vi "AlAs_GaAs_wait_SL_1.vi"(2 "Debug Mode":bool, 3 "Elapsed Time(s)":dbl, 4 "State":enum16{"Edit", "Start", "Run", "End", "Idle"}(ring), 5 "Argument List In":string[](array[string])) -> (0 "Status Out":string, 1 "Argument List Out":string[](array[string]))   [LabVIEW 2011]
doc: "This VI oscillates the flow of Gallium in a square wave according to the \"Period\" and \"Amplitude\" parameters. See the API Programming Guide for more details."
panel:
  in  "tWait2(s)":dbl
  in  "tWait1(s)":dbl
  out "tPeriod(s)":dbl
  in  "periods":dbl
  in  "tGa (s)":dbl
  in  "Ga flow (sccm)":dbl
  in  "tAl (s)":dbl
  in  "Al flow (sccm)":dbl
  in  "Cancel":bool
  in  "OK":bool
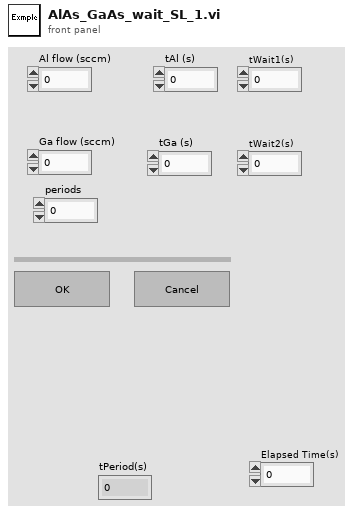
[diagram p1: front panel]
types:
  T1 = enum16{"Discrete", "Continuous", "Instantaneous"}
  T2 = enum32{"Invalid", "Default", "Floating", "Floating/Auto-Hide", "Modal"}
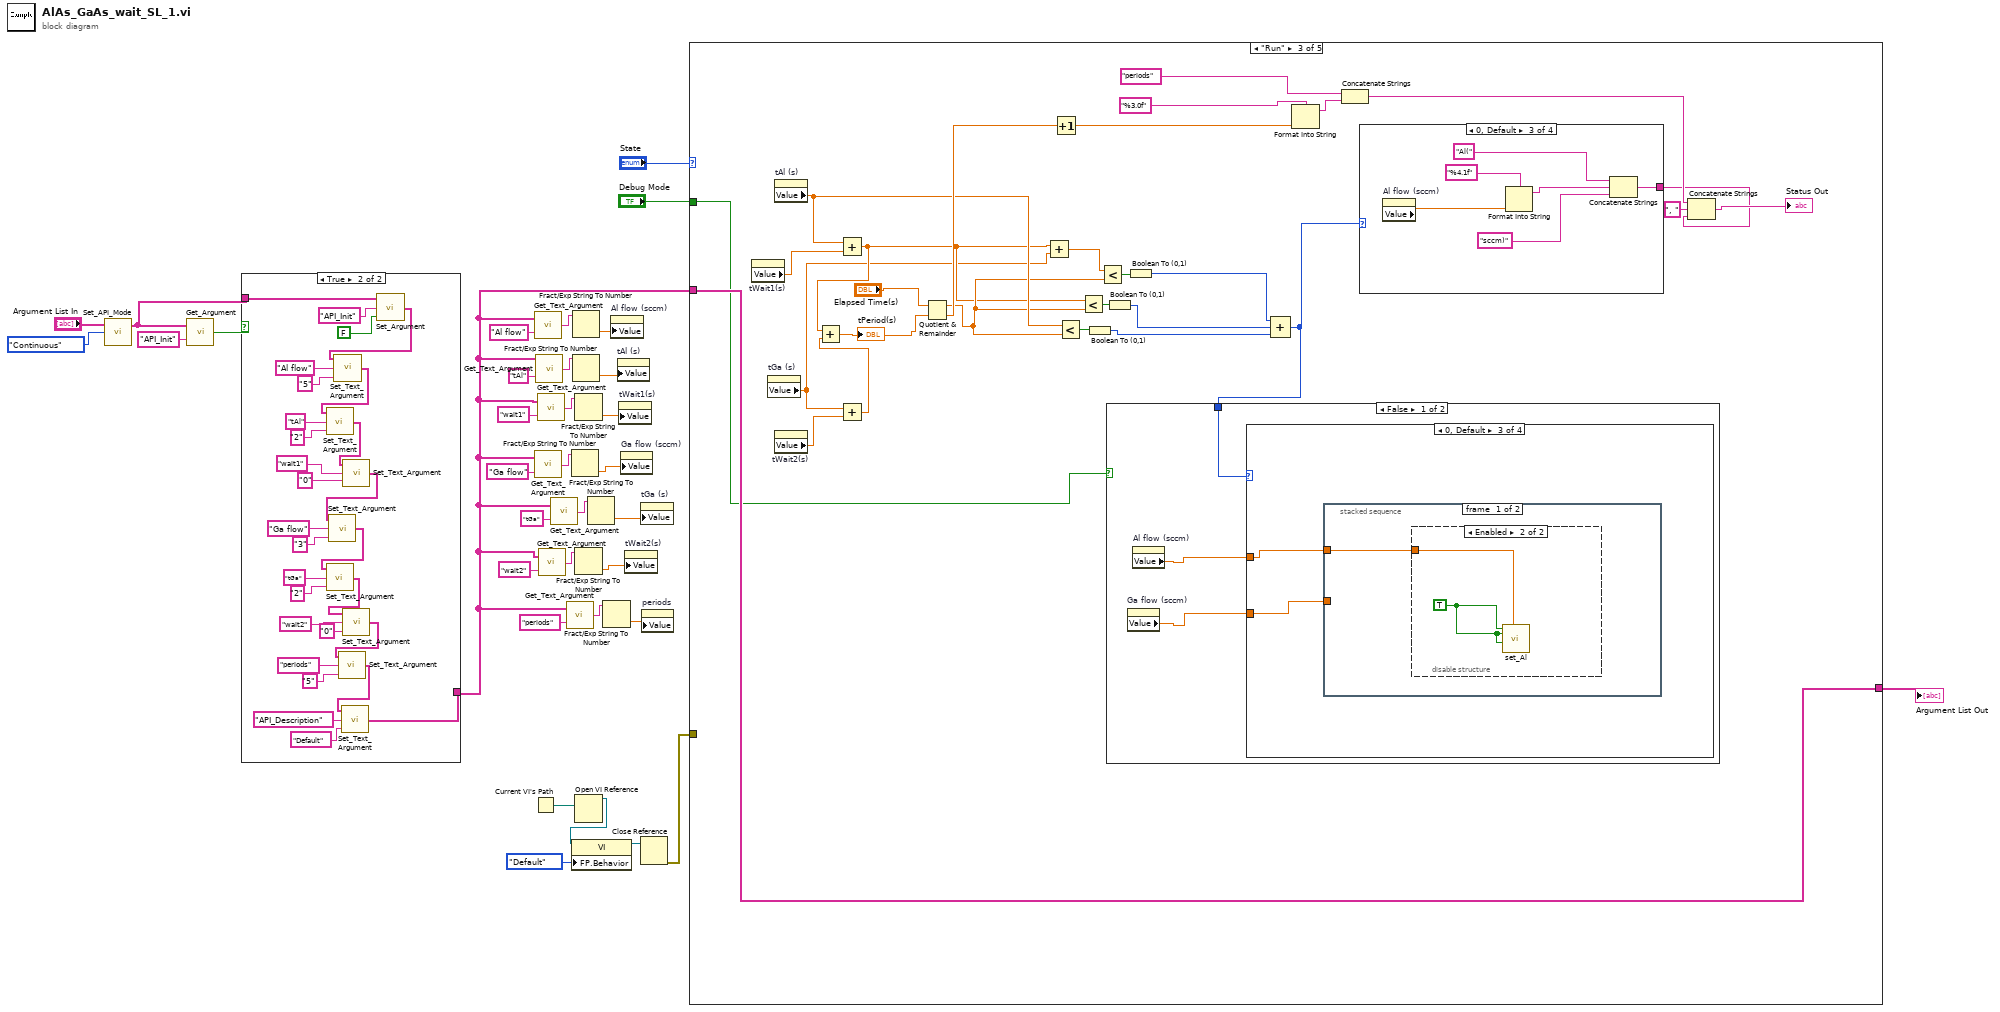
[diagram p0: block diagram]
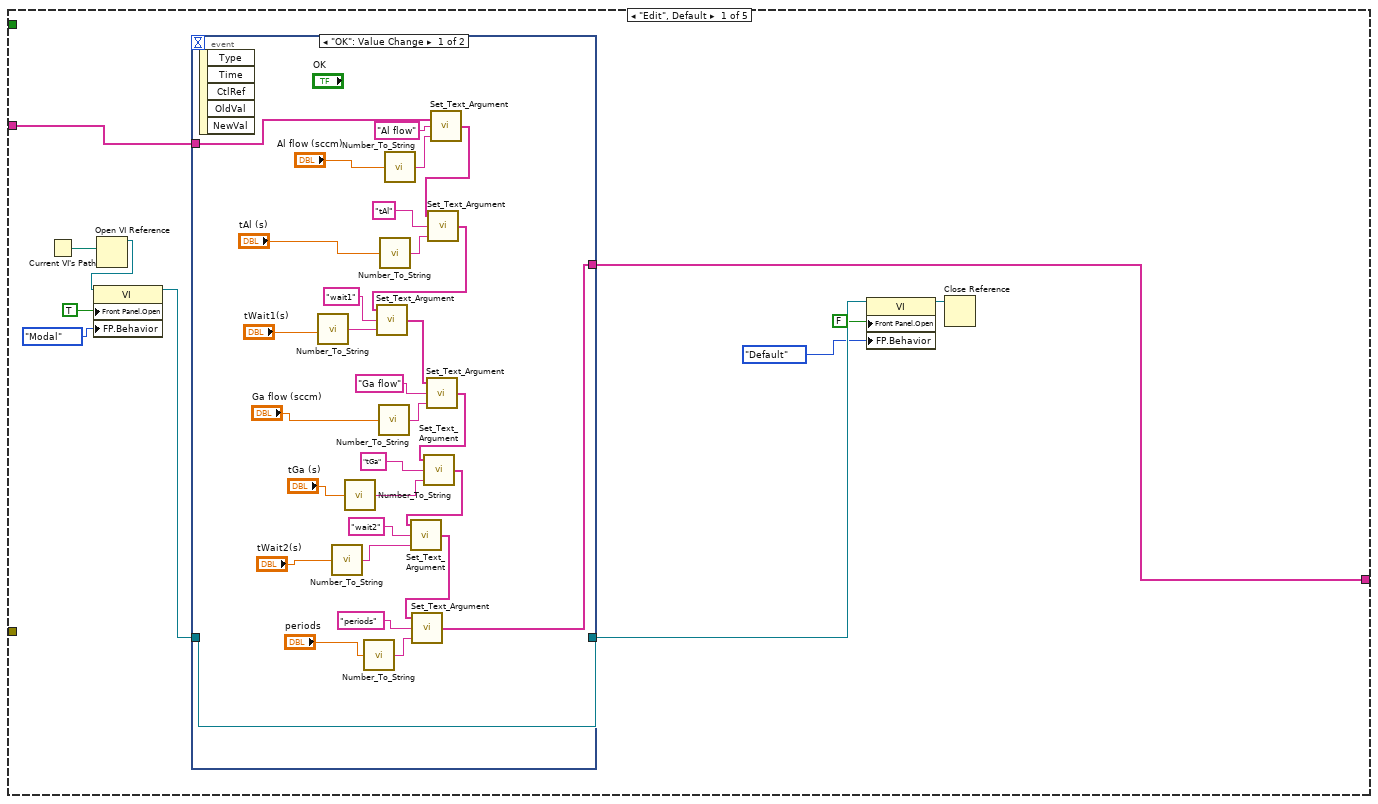
[diagram p3: hidden frame]
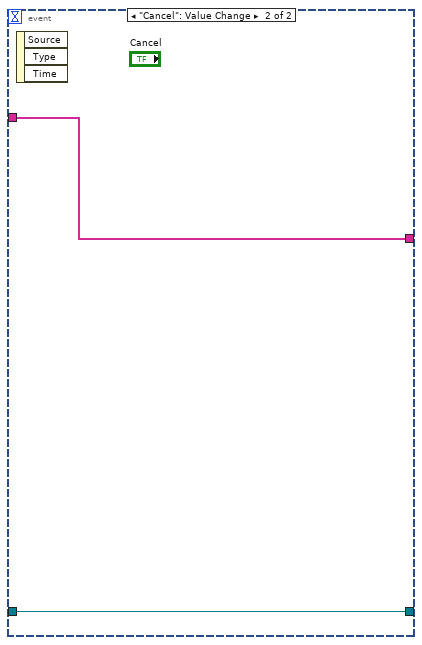
[diagram p4: hidden frame]
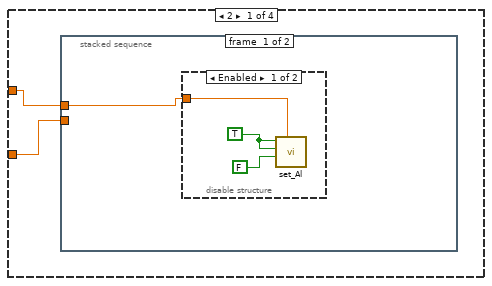
[diagram p6: hidden frame]
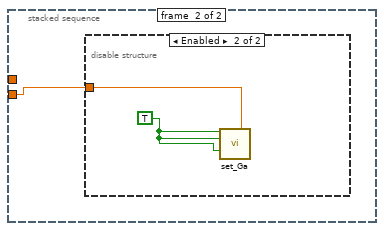
[diagram p8: hidden frame]
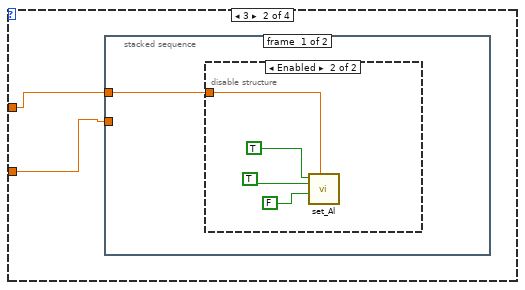
[diagram p10: hidden frame]
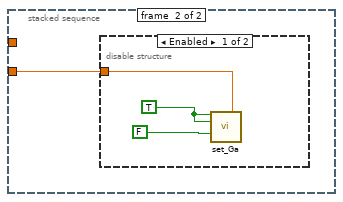
[diagram p12: hidden frame]
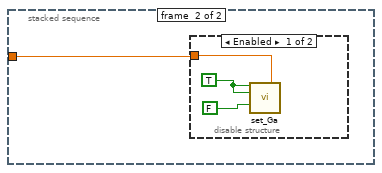
[diagram p15: hidden frame]
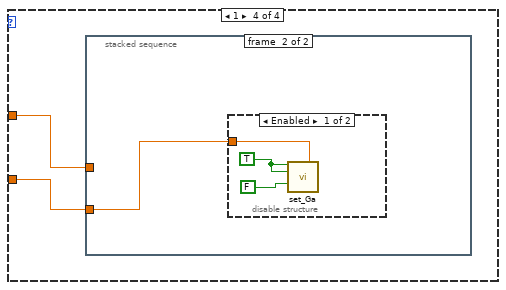
[diagram p17: hidden frame]
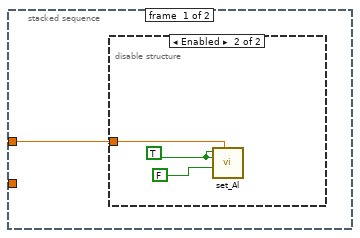
[diagram p18: hidden frame]
diagram:
  n1 = call "Set_API_Mode.vi"("API Mode"=T1."Continuous", "Argument List In"="Argument List In") -> ("Argument List Out"=w22:string[])  [unwired: 2 out]
  n2 = call "Get_Argument.vi"("Argument"="API_Init", "Argument List"=w22) -> ("Enabled"=w23:bool)
  n3 = case shown="True" w23 {
    tunnel: w22 -> [w36 w64]
    tunnel: [w36 w60] -> w3
    frame False {
    }
    frame True {
      n4 = call "Set_Argument.vi"("Enable"=FALSE, "Argument"="API_Init", "Argument List In"=w64) -> ("Argument List Out"=w45:string[])
      n5 = call "Set_Text_Argument.vi"("Text"="5", "Argument"="Al flow", "Argument List In"=w45) -> ("Argument List Out"=w46:string[])
      n6 = call "Set_Text_Argument.vi"("Text"="2", "Argument"="tAl", "Argument List In"=w46) -> ("Argument List Out"=w42:string[])
      n7 = call "Set_Text_Argument.vi"("Text"="0", "Argument"="wait1", "Argument List In"=w42) -> ("Argument List Out"=w41:string[])
      n8 = call "Set_Text_Argument.vi"("Text"="3", "Argument"="Ga flow", "Argument List In"=w41) -> ("Argument List Out"=w47:string[])
      n9 = call "Set_Text_Argument.vi"("Text"="2", "Argument"="tGa", "Argument List In"=w47) -> ("Argument List Out"=w44:string[])
      n10 = call "Set_Text_Argument.vi"("Text"="0", "Argument"="wait2", "Argument List In"=w44) -> ("Argument List Out"=w43:string[])
      n11 = call "Set_Text_Argument.vi"("Text"="5", "Argument"="periods", "Argument List In"=w43) -> ("Argument List Out"=w48:string[])
      n12 = call "Set_Text_Argument.vi"("Text"="Default", "Argument"="API_Description", "Argument List In"=w48) -> ("Argument List Out"=w60:string[])
    }
  }
  n13 = Current VI's Path() -> (path=w31:path)
  n14 = call "Get_Text_Argument.vi"("Argument"="Al flow", "Argument List"=w3) -> ("Text"=w20:string)
  n15 = call "Get_Text_Argument.vi"("Argument"="Ga flow", "Argument List"=w3) -> ("Text"=w17:string)
  n16 = call "Get_Text_Argument.vi"("Argument"="tAl", "Argument List"=w3) -> ("Text"=w19:string)
  n17 = call "Get_Text_Argument.vi"("Argument"="wait1", "Argument List"=w3) -> ("Text"=w6:string)
  n18 = call "Get_Text_Argument.vi"("Argument"="wait2", "Argument List"=w3) -> ("Text"=w2:string)
  n19 = call "Get_Text_Argument.vi"("Argument"="tGa", "Argument List"=w3) -> ("Text"=w15:string)
  n20 = call "Get_Text_Argument.vi"("Argument"="periods", "Argument List"=w3) -> ("Text"=w13:string)
  n21 = Fract/Exp String To Number(string=w17) -> (number=w10:dbl)  [unwired: 4 out]
  n22 = Fract/Exp String To Number(string=w20) -> (number=w12:dbl)  [unwired: 4 out]
  n23 = Fract/Exp String To Number(string=w19) -> (number=w11:dbl)  [unwired: 4 out]
  n24 = Fract/Exp String To Number(string=w6) -> (number=w5:dbl)  [unwired: 4 out]
  n25 = Fract/Exp String To Number(string=w2) -> (number=w1:dbl)  [unwired: 4 out]
  n26 = Open VI Reference(vi path=w31) -> (vi reference=w30:refnum<vi>)  [unwired: 1 in, 5 out]
  n27 = property class="VI"(reference=w30, "FP.Behavior"=T2."Default" ("Front Panel Window:Behavior")) -> (reference out=w28:refnum<vi>)  [unwired: 1 in, 1 out]
  n28 = Fract/Exp String To Number(string=w15) -> (number=w9:dbl)  [unwired: 4 out]
  n29 = Fract/Exp String To Number(string=w13) -> (number=w8:dbl)  [unwired: 4 out]
  n30 = property on="Al flow (sccm)" class="DigNum (strict)"("Value"=w12) -> ()  [unwired: 2 in, 2 out]
  n31 = property on="tAl (s)" class="DigNum (strict)"("Value"=w11) -> ()  [unwired: 2 in, 2 out]
  n32 = property on="tWait1(s)" class="DigNum (strict)"("Value"=w5) -> ()  [unwired: 2 in, 2 out]
  n33 = property on="Ga flow (sccm)" class="DigNum (strict)"("Value"=w10) -> ()  [unwired: 2 in, 2 out]
  n34 = property on="tWait2(s)" class="DigNum (strict)"("Value"=w1) -> ()  [unwired: 2 in, 2 out]
  n35 = property on="tGa (s)" class="DigNum (strict)"("Value"=w9) -> ()  [unwired: 2 in, 2 out]
  n36 = Close Reference(reference=w28) -> (error out=w27:errorcluster)  [unwired: 1 in]
  n37 = property on="periods" class="DigNum (strict)"("Value"=w8) -> ()  [unwired: 2 in, 2 out]
  n38 = case shown="\"Run\"" "State" {
    tunnel: [w75 w108 w136 w194 w195] -> w34
    tunnel: w3 -> [w74 w108 w136 w194 w195]
    tunnel: "Debug Mode" -> [_ _ w110 w193 _]
    tunnel: w27 -> [_ _ _ _ _]
    frame "Edit", Default {
      n39 = Current VI's Path() -> (path=w69:path)
      n40 = Open VI Reference(vi path=w69) -> (vi reference=w68:refnum<vi>)  [unwired: 1 in, 5 out]
      n41 = property class="VI"(reference=w68, "Front Panel.Open"=TRUE ("Front Panel Window:Open"), "FP.Behavior"=T2."Modal" ("Front Panel Window:Behavior")) -> (reference out=w72:refnum<vi>)  [unwired: 1 in, 1 out]
      n42 = event shown="[0] \"OK\": Value Change" {
        selector: _ -> [_ _]
        dyn-events: _ -> [_ _]
        timeout: _ -> [_ _]
        tunnel: w74 -> [w100 w106]
        tunnel: [w90 w106] -> w75
        tunnel: [w104 w107] -> w71
        tunnel: w72 -> [w104 w107]
        event "OK": Value Change {
          n43 = event-data() -> ()  [unwired: 6 out]
          n44 = call "Number_To_String.vi"("Number"="tWait1(s)") -> ("String"=w85:string)
          n45 = call "Number_To_String.vi"("Number"="tWait2(s)") -> ("String"=w79:string)
          n46 = call "Number_To_String.vi"("Number"="tGa (s)") -> ("String"=w94:string)
          n47 = call "Number_To_String.vi"("Number"="periods") -> ("String"=w92:string)
          n48 = call "Number_To_String.vi"("Number"="Ga flow (sccm)") -> ("String"=w96:string)
          n49 = call "Number_To_String.vi"("Number"="tAl (s)") -> ("String"=w101:string)
          n50 = call "Number_To_String.vi"("Number"="Al flow (sccm)") -> ("String"=w97:string)
          n51 = call "Set_Text_Argument.vi"("Text"=w97, "Argument"="Al flow" ("Text"), "Argument List In"=w100) -> ("Argument List Out"=w102:string[])
          n52 = call "Set_Text_Argument.vi"("Text"=w101, "Argument"="tAl", "Argument List In"=w102) -> ("Argument List Out"=w83:string[])
          n53 = call "Set_Text_Argument.vi"("Text"=w85, "Argument"="wait1", "Argument List In"=w83) -> ("Argument List Out"=w82:string[])
          n54 = call "Set_Text_Argument.vi"("Text"=w96, "Argument"="Ga flow", "Argument List In"=w82) -> ("Argument List Out"=w88:string[])
          n55 = call "Set_Text_Argument.vi"("Text"=w94, "Argument"="tGa", "Argument List In"=w88) -> ("Argument List Out"=w81:string[])
          n56 = call "Set_Text_Argument.vi"("Text"=w79, "Argument"="wait2", "Argument List In"=w81) -> ("Argument List Out"=w80:string[])
          n57 = call "Set_Text_Argument.vi"("Text"=w92, "Argument"="periods", "Argument List In"=w80) -> ("Argument List Out"=w90:string[])
        }
        event "Cancel": Value Change {
          n58 = event-data() -> ()  [unwired: 4 out]
        }
      }
      n59 = property class="VI"(reference=w71, "Front Panel.Open"=FALSE ("Front Panel Window:Open"), "FP.Behavior"=T2."Default" ("Front Panel Window:Behavior")) -> (reference out=w65:refnum<vi>)  [unwired: 1 in, 1 out]
      n60 = Close Reference(reference=w65) -> ()  [unwired: 1 in, 1 out]
    }
    frame "Start" {
    }
    frame "Run" {
      n61 = property on="tWait1(s)" class="DigNum (strict)"() -> ("Value"=w111:dbl)  [unwired: 2 in, 2 out]
      n62 = property on="tGa (s)" class="DigNum (strict)"() -> ("Value"=w121:dbl)  [unwired: 2 in, 2 out]
      n63 = property on="tAl (s)" class="DigNum (strict)"() -> ("Value"=w124:dbl)  [unwired: 2 in, 2 out]
      n64 = property on="tWait2(s)" class="DigNum (strict)"() -> ("Value"=w112:dbl)  [unwired: 2 in, 2 out]
      n65 = Add(x=w124, y=w111) -> (x+y=w122:dbl)
      n66 = Add(x=w121, y=w112) -> (x+y=w125:dbl)
      n67 = Add(x=w122, y=w125) -> (x+y=w127:dbl)
      "tPeriod(s)" <- w127
      n68 = Quotient & Remainder(x="Elapsed Time(s)", y=w127) -> (x-y*floor(x/y)=w123:dbl, floor(x/y)=w126:dbl)
      n69 = Add(x=w122, y=w121) -> (x+y=w120:dbl)
      n70 = Increment(x=w126) -> (x+1=w132:dbl)
      n71 = Less?(x=w124, y=w123) -> (x < y?=w119:bool)
      n72 = Less?(x=w122, y=w123) -> (x < y?=w117:bool)
      n73 = Boolean To (0,1)(Boolean=w119) -> (0, 1=w118:i16)
      n74 = Less?(x=w120, y=w123) -> (x < y?=w115:bool)
      n75 = Boolean To (0,1)(Boolean=w117) -> (0, 1=w116:i16)
      n76 = Boolean To (0,1)(Boolean=w115) -> (0, 1=w114:i16)
      n77 = Compound Arithmetic op=ADD(w114, w116, w118) -> (w109:i16)
      n78 = case shown="False" w110 {
        tunnel: w109 -> [w139 _]
        frame False {
          n79 = property on="Ga flow (sccm)" class="DigNum (strict)"() -> ("Value"=w137:dbl)  [unwired: 2 in, 2 out]
          n80 = property on="Al flow (sccm)" class="DigNum (strict)"() -> ("Value"=w138:dbl)  [unwired: 2 in, 2 out]
          n81 = case shown="0, Default" w139 {
            tunnel: w138 -> [w141 w150 w161 w170]
            tunnel: w137 -> [w140 w149 w160 w169]
            frame 2 {
              n82 = stacked-sequence {
                tunnel: w141 -> [w142 _]
                tunnel: w140 -> [_ w146]
                frame #0 {
                  n83 = disable-structure shown="Enabled" {
                    disable-tunnel: w142 -> [w143 _]
                    frame Enabled {
                      w145 = TRUE ("Ga Active")
                      n84 = call "set_Al.vi"("Aluminum Flow"=w143, "Al Run"=FALSE, "Al Bubbler"=w145, "Al Active"=w145) -> ()  [unwired: 6 in]
                    }
                    frame Disabled {
                    }
                  }
                }
                frame #1 {
                  n85 = disable-structure shown="Enabled" {
                    disable-tunnel: w146 -> [_ w148]
                    frame Disabled {
                    }
                    frame Enabled {
                      w147 = TRUE ("Ga Active")
                      n86 = call "set_Ga.vi"("Ga Active"=w147, "Ga Flow 1"=w148, "Ga Bubbler"=w147, "Ga Run"=w147) -> ()  [unwired: 12 in]
                    }
                  }
                }
              }
            }
            frame 3 {
              n87 = stacked-sequence {
                tunnel: w150 -> [w151 _]
                tunnel: w149 -> [_ w156]
                frame #0 {
                  n88 = disable-structure shown="Enabled" {
                    disable-tunnel: w151 -> [_ w152]
                    frame Disabled {
                    }
                    frame Enabled {
                      n89 = call "set_Al.vi"("Aluminum Flow"=w152, "Al Run"=FALSE, "Al Bubbler"=TRUE, "Al Active"=TRUE) -> ()  [unwired: 6 in]
                    }
                  }
                }
                frame #1 {
                  n90 = disable-structure shown="Enabled" {
                    disable-tunnel: w156 -> [w157 _]
                    frame Enabled {
                      w158 = TRUE ("Ga Active")
                      n91 = call "set_Ga.vi"("Ga Active"=w158, "Ga Flow 1"=w157, "Ga Bubbler"=w158, "Ga Run"=FALSE) -> ()  [unwired: 4 in, 8 out]
                    }
                    frame Disabled {
                    }
                  }
                }
              }
            }
            frame 0, Default {
              n92 = stacked-sequence {
                tunnel: w161 -> [w162 _]
                tunnel: w160 -> [_ w165]
                frame #0 {
                  n93 = disable-structure shown="Enabled" {
                    disable-tunnel: w162 -> [_ w164]
                    frame Disabled {
                    }
                    frame Enabled {
                      w163 = TRUE ("Al Active")
                      n94 = call "set_Al.vi"("Aluminum Flow"=w164, "Al Run"=w163, "Al Bubbler"=w163, "Al Active"=w163) -> ()  [unwired: 6 in]
                    }
                  }
                }
                frame #1 {
                  n95 = disable-structure shown="Enabled" {
                    disable-tunnel: w165 -> [w166 _]
                    frame Enabled {
                      w167 = TRUE ("Ga Active")
                      n96 = call "set_Ga.vi"("Ga Active"=w167, "Ga Flow 1"=w166, "Ga Bubbler"=w167, "Ga Run"=FALSE) -> ()  [unwired: 4 in, 8 out]
                    }
                    frame Disabled {
                    }
                  }
                }
              }
            }
            frame 1 {
              n97 = stacked-sequence {
                tunnel: w169 -> [_ w175]
                tunnel: w170 -> [w171 _]
                frame #0 {
                  n98 = disable-structure shown="Enabled" {
                    disable-tunnel: w171 -> [_ w173]
                    frame Disabled {
                    }
                    frame Enabled {
                      w172 = TRUE ("Al Bubbler")
                      n99 = call "set_Al.vi"("Aluminum Flow"=w173, "Al Run"=FALSE, "Al Bubbler"=w172, "Al Active"=w172) -> ()  [unwired: 6 in]
                    }
                  }
                }
                frame #1 {
                  n100 = disable-structure shown="Enabled" {
                    disable-tunnel: w175 -> [w176 _]
                    frame Enabled {
                      w177 = TRUE ("Ga Active")
                      n101 = call "set_Ga.vi"("Ga Active"=w177, "Ga Flow 1"=w176, "Ga Bubbler"=w177, "Ga Run"=FALSE) -> ()  [unwired: 4 in, 8 out]
                    }
                    frame Disabled {
                    }
                  }
                }
              }
            }
          }
        }
        frame True {
        }
      }
      n102 = Format Into String(format string="%3.0f", w132) -> (resulting string=w133:string)  [unwired: 2 in, 1 out]
      n103 = Concatenate Strings("periods" ("string"), w133) -> (w130:string)
      n104 = case shown="0, Default" w109 {
        tunnel: [w179 "wait" w186 "wait"] -> w113
        frame 2 {
          n105 = property on="Ga flow (sccm)" class="DigNum (strict)"() -> ("Value"=w180:dbl)  [unwired: 2 in, 2 out]
          n106 = Format Into String(format string="%4.2f", w180) -> (resulting string=w183:string)  [unwired: 2 in, 1 out]
          n107 = Concatenate Strings("Ga(" ("string"), w183, "sccm)" ("string")) -> (w179:string)
        }
        frame 3 {
        }
        frame 0, Default {
          n108 = property on="Al flow (sccm)" class="DigNum (strict)"() -> ("Value"=w187:dbl)  [unwired: 2 in, 2 out]
          n109 = Format Into String(format string="%4.1f", w187) -> (resulting string=w189:string)  [unwired: 2 in, 1 out]
          n110 = Concatenate Strings("Al(" ("string"), w189, "sccm)" ("string")) -> (w186:string)
        }
        frame 1 {
        }
      }
      n111 = Concatenate Strings(w130, ", " ("string"), w113) -> (→"Status Out":string)
    }
    frame "End" {
      n112 = case shown="False" w193 {
        frame False {
        }
        frame True {
        }
      }
    }
    frame "Idle" {
    }
  }
  "Argument List Out" <- w34
